vi "rad_Deploy All Bitfiles.vi"(5 "Password":string, 8 "error in (no error)":errorcluster, 9 "FPGA Properties":T1, 10 "Unzipped files":path[](array[path]), 11 "Target settings in":T3={"Hostname"="", "Serial number"="", "Product name"="", "Product code"=0, "System status"="", "Credential type"=enum."None/Unlocked", "User added?"=FALSE, "Primary NIC"={"MAC address"="", "IP Address Request Mode"=2, "IP address"="", "Subnet mask"="", "Gateway"="", "DNS server"=""}} {"Primary NIC"."IP Address Request Mode" items=["Static"=1, "DHCP/Link-Local"=2, "Link-Local Only"=4, "DHCP Only"=8]}) -> (0 "error out":errorcluster)   [LabVIEW 2020]
uses:
  <vilib>/nisyscfg/nisyscfg.lvlib
  <resource>/objmgr/niflexrioatomicsae.rc
  <vilib>/nisyscfg/Find Hardware.vi
  <vilib>/nisyscfg/Close (System).vi
  <vilib>/nisyscfg/Upgrade Firmware (File).vi
  <vilib>/nisyscfg/Close (Hardware).vi
  <vilib>/nisyscfg/Close (Filter).vi
  TypeDefs/rad_FPGA Flash Properties.ctl
  TypeDefs/rad_FPGA Properties.ctl
  Targets/TypeDefs/rad_Target Information.ctl
  Targets/TypeDefs/rad_Target Network Settings.ctl
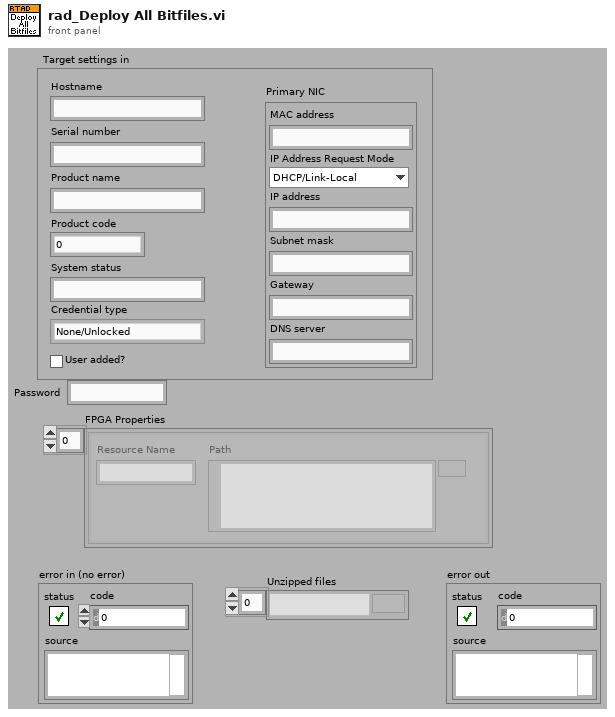
[diagram p1: front panel]
types:
  T1 = typedef "rad_FPGA Properties.ctl" = T2[]
  T2 = typedef "rad_FPGA Flash Properties.ctl" = cluster{"Resource Name":string, "Path":path}
  T3 = typedef "rad_Target Information.ctl" = cluster{"Hostname":string, "Serial number":string, "Product name":string, "Product code":i32, "System status":string, "Credential type":enum16{"None/Unlocked", "FTP Password", "NIAuth Credentials"}, "User added?":bool, "Primary NIC":T4}
  T4 = typedef "rad_Target Network Settings.ctl" = cluster{"MAC address":string, "IP Address Request Mode":i32, "IP address":string, "Subnet mask":string, "Gateway":string, "DNS server":string}
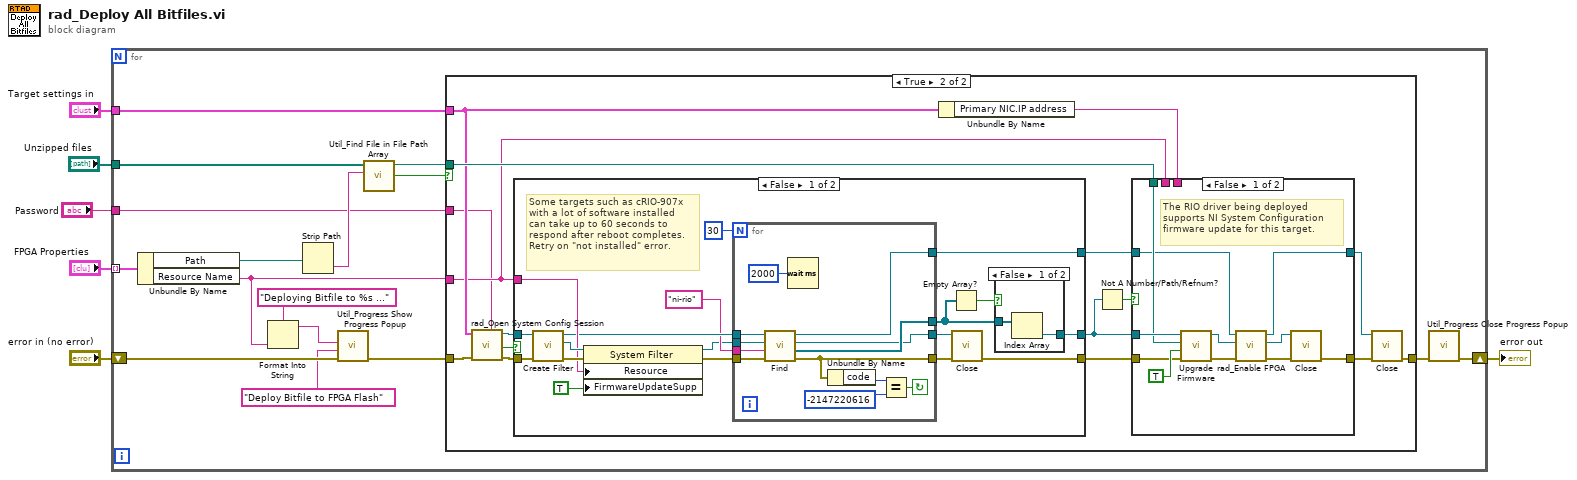
[diagram p0: block diagram]
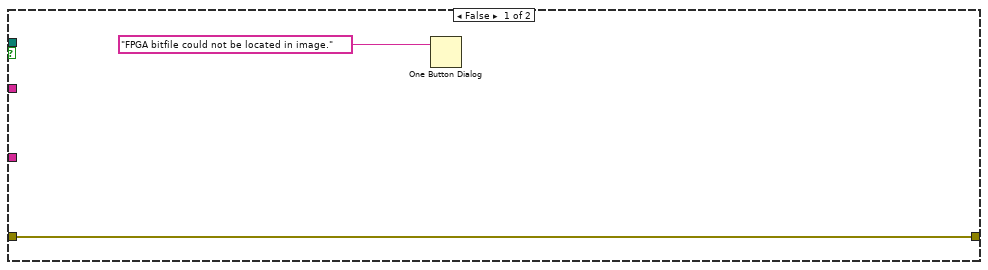
[diagram p2: hidden frame]
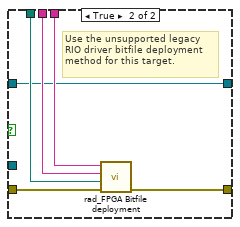
[diagram p3: hidden frame]
diagram:
  n1 = for {
    shift-right: [w16] -> w5
    shift-left: "error in (no error)" -> [w19]
    tunnel: "FPGA Properties" -> [w20] mode=indexing
    tunnel: "Unzipped files" -> [w8]
    tunnel: "Target settings in" -> [w12]
    tunnel: "Password" -> [w7]
    n2 = Unbundle By Name(w20) -> ("Path"=w9:path, "Resource Name"=w11:string)
    n3 = Format Into String(format string="Deploying Bitfile to %s ..." ("Message"), w11) -> (resulting string=w22:string)  [unwired: 2 in, 1 out]
    n4 = Strip Path(path=w9) -> (name=w21:string)  [unwired: 1 out]
    n5 = call "Util_Progress Show Progress Popup.vi"("error in (no error)"=w19, "Title"="Deploy Bitfile to FPGA Flash", "Message"=w22) -> ("error out"=w18:errorcluster)  [unwired: 8 in]
    n6 = call "Util_Find File in File Path Array.vi"("Target file"=w21, "Files"=w8) -> ("Found?"=w15:bool, "Output Path"=w10:path)  [unwired: 7 in, 1 out]
    n7 = case shown="True" w15 {
      tunnel: w12 -> [_ w32]
      tunnel: w18 -> [w24 w40]
      tunnel: [w24 w27] -> w17
      tunnel: w11 -> [_ w30]
      tunnel: w10 -> [_ w33]
      tunnel: w7 -> [_ w25]
      frame False {
        n8 = One Button Dialog(message="FPGA bitfile could not be located in image.") -> ()  [unwired: 1 in, 1 out]
      }
      frame True {
        n9 = call "rad_Open System Config Session.vi"("Password"=w25, "error in (no error)"=w40, "Target settings"=w32) -> ("error out"=w39:errorcluster, "Cancelled"=w37:bool, "Session out"=w38:refnum<k21>)  [unwired: 5 in, 1 out]
        n10 = case shown="False" w37 {
          tunnel: w39 -> [w72 w90]
          tunnel: w38 -> [w73 _]
          tunnel: [w61 w90] -> w34
          tunnel: w30 -> [w71 _]
          tunnel: [w60 _] -> w35
          tunnel: [w59 _] -> w29
          frame False {
            # "Some targets such as cRIO-907x\nwith a lot of software installed\ncan take up to 60 seconds to\nrespond after reboot completes.\nRetry on \"not installed\" error."
            n11 = call <vilib>:"Create Filter.vi"("error in (no error)"=w72, "Session in"=w73) -> ("error out"=w75:errorcluster, "Filter out"=w74:refnum<k20>, "Session out"=w69:refnum<k21>)  [unwired: 7 in]
            n12 = property class="System Filter"(reference=w74, error in=w75, "Resource"=w71, "FirmwareUpdateSupp"=TRUE ("Devices & Chassis:Supports Firmware Update")) -> (reference out=w67:refnum<k20>, error out=w70:errorcluster)
            n13 = for {
              N: 30 -> [_]
              tunnel: w70 -> [w87]
              tunnel: w69 -> [w86]
              tunnel: "ni-rio" ("experts") -> [w85]
              tunnel: w67 -> [w84]
              tunnel: [w83] -> w64
              tunnel: [w82] -> w63
              tunnel: [w79] -> w62
              tunnel: [w81] -> w59
              stop <- w77 continue-if-true
              n14 = call-poly <vilib>:"Find.vi"("error in (no error)"=w87, "Experts"=w85, "Filter in"=w84, "Session in"=w86) -> ("error out"=w79:errorcluster, "Resources out"=w83:refnum<k20>[], "Filter out"=w82:refnum<k20>, "Session out"=w81:refnum<k21>)  [unwired: 4 in]
              n15 = Wait (ms)(milliseconds to wait=u32 2000) -> ()  [unwired: 1 out]
              n16 = Unbundle By Name(w79) -> ("code"=w78:i32)
              n17 = Equal?(x=w78, y=-2147220616) -> (x = y?=w77:bool)
            }
            n18 = Empty Array?(array=w64) -> (empty?=w65:bool)
            n19 = call-poly <vilib>:"Close.vi"("error in (no error)"=w62, "Filter in"=w63) -> ("error out"=w61:errorcluster)  [unwired: 9 in]
            n20 = case shown="False" w65 {
              tunnel: w64 -> [w89 _]
              tunnel: [w88 _] -> w60
              frame False {
                n21 = Index Array(array=w89) -> (element=w88:refnum<k20>)  [unwired: 1 in]
              }
              frame True {
              }
            }
          }
          frame True {
          }
        }
        n22 = Unbundle By Name(w32) -> ("Primary NIC.IP address"=w31:string)
        n23 = Not A Number/Path/Refnum?(number/path/refnum=w35) -> (NaN/Path/Refnum?=w36:bool)
        n24 = case shown="False" w36 {
          tunnel: [w50 w55] -> w28
          tunnel: w35 -> [w49 _]
          tunnel: w34 -> [w48 w56]
          tunnel: w33 -> [w47 w54]
          tunnel: w31 -> [_ w57]
          tunnel: w30 -> [_ w53]
          tunnel: w29 -> [w45 w52]
          tunnel: [w41 w52] -> w26
          frame False {
            # "The RIO driver being deployed\nsupports NI System Configuration\nfirmware update for this target."
            n25 = call-poly <vilib>:"Upgrade Firmware.vi"("error in (no error)"=w48, "Always Overwrite (F)"=TRUE ("always overwrite (F)"), "Firmware File"=w47, "Resource in"=w49) -> ("error out"=w44:errorcluster, "Resource out"=w46:refnum<k20>)  [unwired: 4 in, 2 out]
            n26 = call "rad_Enable FPGA.vi"("error in (no error)"=w44, "device in"=w46, "session in"=w45) -> ("error out"=w42:errorcluster, "device out"=w43:refnum<k20>, "session out"=w41:refnum<k21>)  [unwired: 6 in]
            n27 = call-poly <vilib>:"Close.vi"("error in (no error)"=w42, "Resource in"=w43) -> ("error out"=w50:errorcluster)  [unwired: 9 in]
          }
          frame True {
            # "Use the unsupported legacy\nRIO driver bitfile deployment\nmethod for this target."
            n28 = call "rad_FPGA Bitfile deployment.vi"("error in (no error)"=w56, "Bitfile path"=w54, "Resource Name"=w53, "IP Address"=w57) -> ("error out"=w55:errorcluster)  [unwired: 7 in]
          }
        }
        n29 = call-poly <vilib>:"Close.vi"("error in (no error)"=w28, "Session in"=w26) -> ("error out"=w27:errorcluster)  [unwired: 9 in]
      }
    }
    n30 = call "Util_Progress Close Progress Popup.vi"("error in (no error)"=w17) -> ("error out"=w16:errorcluster)  [unwired: 10 in]
  }
  "error out" <- w5
